vi "Initialize Global DaisyChain.vi"(0 "System no.":i32=1 min=1 step=1, 5 "error in":errorcluster) -> (19 "error out":errorcluster)   [LabVIEW 2020]
doc: "This VI initializes Global DaisyChain according to the given System no. \n\nE-709: Only supported if E-709 is used inside C-867K012/K013."
uses:
  ProgramData/PI/LabVIEW/Low Level/Communication.llb/Global DaisyChain.vi
panel:
  # "This vi initializes Global DaisyChain\naccording to the given system no."
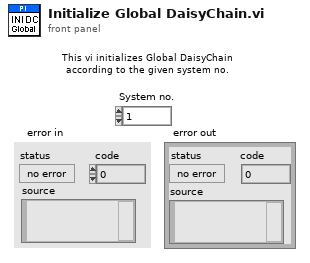
[diagram p1: front panel]
types:
  T1 = cluster{"No. of devices":i32, "Port ID":i32, "Devices":string[], "Description":string}[]
  T2 = cluster{"No. of devices":i32, "Port ID":i32, "Devices":string[], "Description":string}
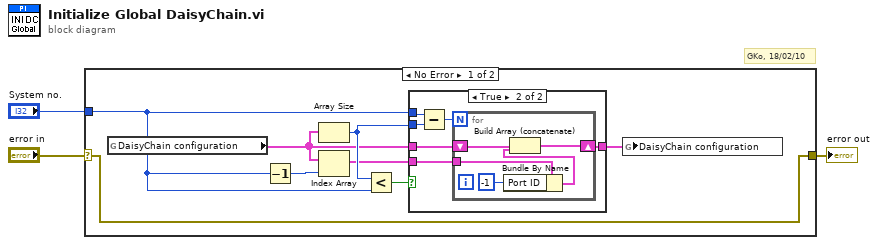
[diagram p0: block diagram]
diagram:
  # "GKo, 18/02/10"
  n1 = case shown="No Error" "error in" {
    selector: "error in" -> [w7 w24]
    tunnel: "System no." -> [w10 _]
    tunnel: [w7 w24] -> w1
    frame No Error {
      n2 = global read "Global DaisyChain.vi" "DaisyChain configuration"() -> (w6:T1)
      n3 = Decrement(x=w10) -> (x-1=w4:i32)
      n4 = Array Size(array=w6) -> (size(s)=w9:i32)
      n5 = Index Array(array=w6, index=w4) -> (element=w8:T2)
      n6 = Less?(x=w9, y=w10) -> (x < y?=w11:bool)
      n7 = case shown="True" w11 {
        tunnel: w10 -> [_ w17]
        tunnel: w9 -> [_ w16]
        tunnel: w6 -> [w12 w15]
        tunnel: w8 -> [_ w14]
        tunnel: [w12 w13] -> w5
        frame False {
        }
        frame True {
          n8 = Subtract(x=w17, y=w16) -> (x-y=w18:i32)
          n9 = for {
            N: w18 -> [_]
            shift-right: [w23] -> w13
            shift-left: w15 -> [w22]
            tunnel: w14 -> [w21]
            n10 = Bundle By Name(cluster=w21, "Port ID"=-1) -> (w19:T2)
            n11 = Build Array (concatenate)(w22, w19) -> (w23:T1)
          }
        }
      }
      n12 = global write "Global DaisyChain.vi" "DaisyChain configuration"(w5) -> ()
    }
    frame Error {
    }
  }
  "error out" <- w1
